vi "Load-configuration-with-dialog.vi"(8 "error in (no error)":errorcluster, 11 "Object ref in":T1) -> (0 "error out":errorcluster, 3 "Object ref out":T1)   [LabVIEW 2013, in "HardwareCharacterization.lvlib" / "HC-Main.lvclass"]
uses:
  HC-Main.lvclass
  Object-reference.ctl
  HC-Main.lvclass/HC-Main.ctl
  UI/Control-names.ctl
  Configuration-data.ctl
  Options.ctl
  Application-status.ctl
  Read UI.vi
  Read Status.vi
  Read Base path.vi
  <vilib>/Utility/xml.llb/Read From XML File(string).vi
  UI/Set-control-enable-single.vi
  UI/HC-UI.lvclass
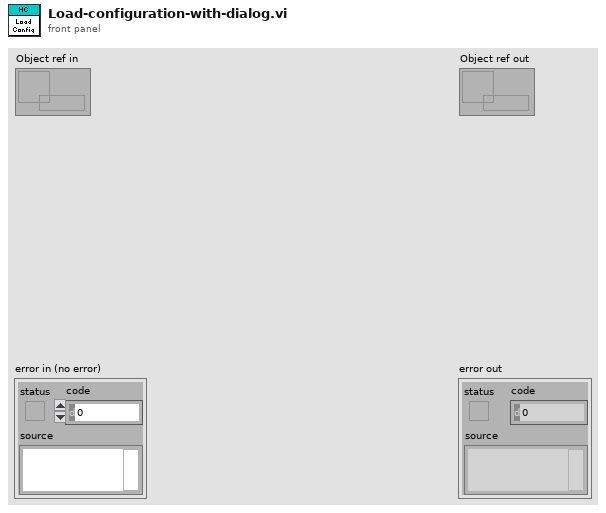
[diagram p1: front panel]
types:
  T1 = typedef "HardwareCharacterization.lvlib/HC-Main.lvclass/Object-reference.ctl" = refnum<data-value>
  T2 = typedef "HardwareCharacterization.lvlib/HC-Main.lvclass/Configuration-data.ctl" = cluster{"Options":T3}
  T3 = typedef "HardwareCharacterization.lvlib/HC-Main.lvclass/Options.ctl" = cluster{"Option 1":bool}
  T4 = typedef "HardwareCharacterization.lvlib/HC-UI.lvclass/Control-names.ctl" = enum16{"Help", "Status", "Load configuration", "Save configuration", "Activate", "Start", "Stop", "Options"}
  T5 = typedef "HardwareCharacterization.lvlib/HC-Main.lvclass/Application-status.ctl" = enum16{"Idle", "Initialized", "Configured", "Activated", "Started", "Paused", "Stopped", "Reset", "Error", "Exited"}
  T6 = typedef "HardwareCharacterization.lvlib/HC-UI.lvclass/Panes-reference.ctl" = refnum<data-value>
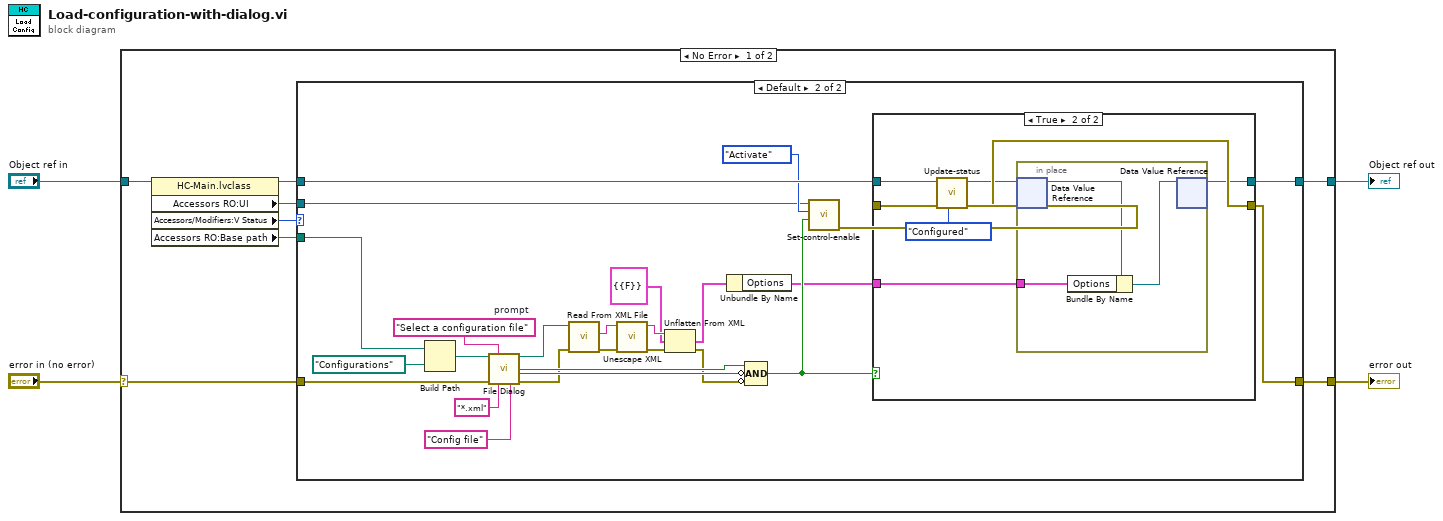
[diagram p0: block diagram]
diagram:
  n1 = case shown="No Error" "error in (no error)" {
    selector: "error in (no error)" -> [w12 w54]
    tunnel: [w8 w54] -> w3
    tunnel: [w7 w53] -> w1
    tunnel: "Object ref in" -> [w11 w53]
    frame No Error {
      n2 = property class="HC-Main.lvclass"(reference=w11) -> (reference out=w9:T1, "Accessors RO:UI"=w10:T6, "Accessors/Modifiers:V Status"=w6:T5, "Accessors RO:Base path"=w5:path)  [unwired: 1 in, 1 out]
      n3 = case shown="Default" w6 {
        tunnel: w12 -> [w14 w38]
        tunnel: w10 -> [_ w16]
        tunnel: w9 -> [w13 w32]
        tunnel: [w14 w31] -> w8
        tunnel: [w13 w21] -> w7
        tunnel: w5 -> [_ w19]
        frame "Activated".."Paused" {
        }
        frame Default {
          w40 = "Select a configuration file"  # prompt
          n4 = Build Path(base path=w19, name or relative path=path "Configurations") -> (appended path=w18:path)
          n5 = call "File Dialog"("start path"=w18, "prompt"=w40, "error in"=w38, "pattern (all files)"="*.xml", "pattern label"="Config file") -> ("selected path"=w29:path, "exists"=w36:bool, "cancelled"=w35:bool, "error out"=w23:errorcluster)  [unwired: 7 in]
          n6 = call-poly <vilib>:"Read From XML File.vi"("error in (no error)"=w23, "XML File Path"=w29) -> ("error out"=w28:errorcluster, "XML Elements"=w27:string)  [unwired: 7 in, 1 out]
          n7 = call <vilib>:"Unescape XML.vi"("error in (no error)"=w28, "XML String In"=w27) -> ("error out"=w26:errorcluster, "XML String Out"=w25:string)  [unwired: 8 in]
          n8 = Unflatten From XML(xml string=w25, type=T2 {"Options"={"Option 1"=FALSE}} ("Configuration data"), error in (no error)=w26) -> (value=w17:T2, error out=w22:errorcluster)
          n9 = Unbundle By Name(w17) -> ("Options"=w15:T3)
          n10 = Compound Arithmetic op=AND(w36, invert w35, invert w22) -> (w34:bool)
          n11 = call-poly "Set-control-enable.vi"("Enable?"=w34, "Control name"=Control-names."Activate", "Panes in"=w16) -> ("error out"=w33:errorcluster)  [unwired: 7 in, 1 out]
          n12 = case shown="True" w34 {
            tunnel: [w41 w49] -> w31
            tunnel: [w42 w44] -> w21
            tunnel: w33 -> [w41 w46]
            tunnel: w32 -> [w42 w47]
            tunnel: w15 -> [_ w43]
            frame False {
            }
            frame True {
              n13 = call "Update-status.vi"("Status"=Application-status."Configured", "error in (no error)"=w46, "Object ref in"=w47) -> ("error out"=w49:errorcluster, "Object ref out"=w45:T1)  [unwired: 7 in]
              n14 = in-place {
                in-place-border: w43 -> [w50]
                n15 = in-place-dvr #1(w45) -> (w52:refnum<class "HC-Main.lvclass">)  [unwired: 1 out]
                n16 = Bundle By Name(cluster=w52, "Options"=w50) -> (w51:refnum<class "HC-Main.lvclass">)
                n17 = in-place-dvr #1(w51) -> (w44:T1)  [unwired: 1 out]
              }
            }
          }
        }
      }
    }
    frame Error {
    }
  }
  "error out" <- w3
  "Object ref out" <- w1
